vi "Focus Grid Chooser.vi"(10 "SEM Scan Parameters":T2={"X size (um)"=80.0, "Y size (um)"=80.0, "X center (um)"=0.0, "Y center (um)"=0.0, "X size (V)"=3.7333333333333334, "X size auto"=TRUE, "X stig"=[[0.0]], "Y stig"=[[0.0]], "X aln"=[[0.0]], "Y aln"=[[0.0]], "Scan rate (Hz)"=10000000, "Oversampling"=5, "Oversampling auto"=TRUE, "Frame line rampdown ratio"=0.1, "Pixel size (nm)"=8.0, "WD (mm)"=[[3.0]], "X tiles"=1, "Y tiles"=1, "Overlap (um)"=2.0, "Interlaced"=TRUE, "dX (um)"=[0.0], "dY (um)"=[0.0], "Frames"=1} {"dY (um)" format="%.1f"; "dX (um)" format="%.1f"; "Frames" min=1 step=1; "WD (mm)" step=0.001 format="%.4f"; "Y aln" format="%.1f"; "X aln" format="%.1f"; "Y stig" format="%.1f"; "X stig" format="%.1f"; "Overlap (um)" min=0; "Y tiles" min=1; "X tiles" min=1; "X size (um)" format="%.2f"; "Y size (um)" format="%.2f"; "Frame line rampdown ratio" min=0 max=1 step=0.05 format="%.2g"; "X center (um)" step=1 format="%.3f"; "Y center (um)" step=1 format="%.3f"; "X size (V)" format="%_4g"; "Scan rate (Hz)" max=4000000 step=100000 format="%.2e"}, 11 "Focus Index Options":T1={"Keep aspect ratio"=FALSE, "Show Focus Index"=TRUE, "Focus Index primary grid center"=TRUE, "X Grids"=[[1]], "Y Grids"=[[1]], "Primary X index"=[[1]], "Primary Y index"=[[1]]} {"Y Grids" step=2; "X Grids" step=2}) -> (3 "Focus Index Options Out":T1={"Keep aspect ratio"=FALSE, "Show Focus Index"=TRUE, "Focus Index primary grid center"=TRUE, "X Grids"=[[1]], "Y Grids"=[[1]], "Primary X index"=[[1]], "Primary Y index"=[[1]]} {"Y Grids" step=2; "X Grids" step=2})   [LabVIEW 2018]
panel:
  in  "Centered":bool
  out "X Prmry out":u8[][](array[numeric])
  out "Y Prmry out":u8[][](array[numeric])
  out "Tile Y":i32
  out "Tile X":i32
  in  "Tile Grid":bool[][](array[boolean])=[[TRUE, FALSE, FALSE, FALSE, FALSE], [FALSE, FALSE, FALSE, FALSE, FALSE]] caption="Block Face Tile Grid"
  in  "Finished":bool
  out "Y Prmry":u8
  out "X Prmry":u8
  in  "Nx Grids":u8=1 min=1 step=1
  in  "Ny Grids":u8=1 min=1 step=1
  in  "PF Grid":bool[][](array[boolean]) caption="Tile's Primary-Focus Grid"
  # "Grids"
  # "Primary"
  # "Grids"
  # "Primary"
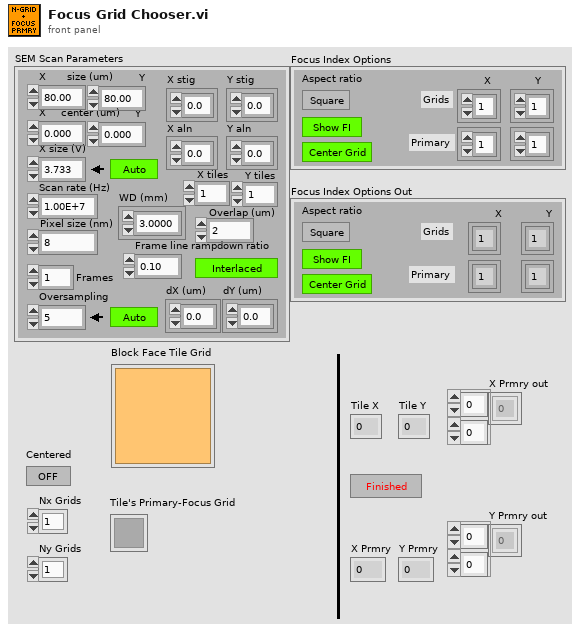
[diagram p1: front panel]
types:
  T1 = cluster{"Keep aspect ratio":bool, "Show Focus Index":bool, "Focus Index primary grid center":bool, "X Grids":u8[][], "Y Grids":u8[][], "Primary X index":u8[][], "Primary Y index":u8[][]}
  T2 = cluster{"X size (um)":sgl, "Y size (um)":sgl, "X center (um)":sgl, "Y center (um)":sgl, "X size (V)":dbl, "X size auto":bool, "X stig":sgl[][], "Y stig":sgl[][], "X aln":sgl[][], "Y aln":sgl[][], "Scan rate (Hz)":u32, "Oversampling":u32, "Oversampling auto":bool, "Frame line rampdown ratio":sgl, "Pixel size (nm)":sgl, "WD (mm)":sgl[][], "X tiles":u8, "Y tiles":u8, "Overlap (um)":sgl, "Interlaced":bool, "dX (um)":sgl[], "dY (um)":sgl[], "Frames":u8}
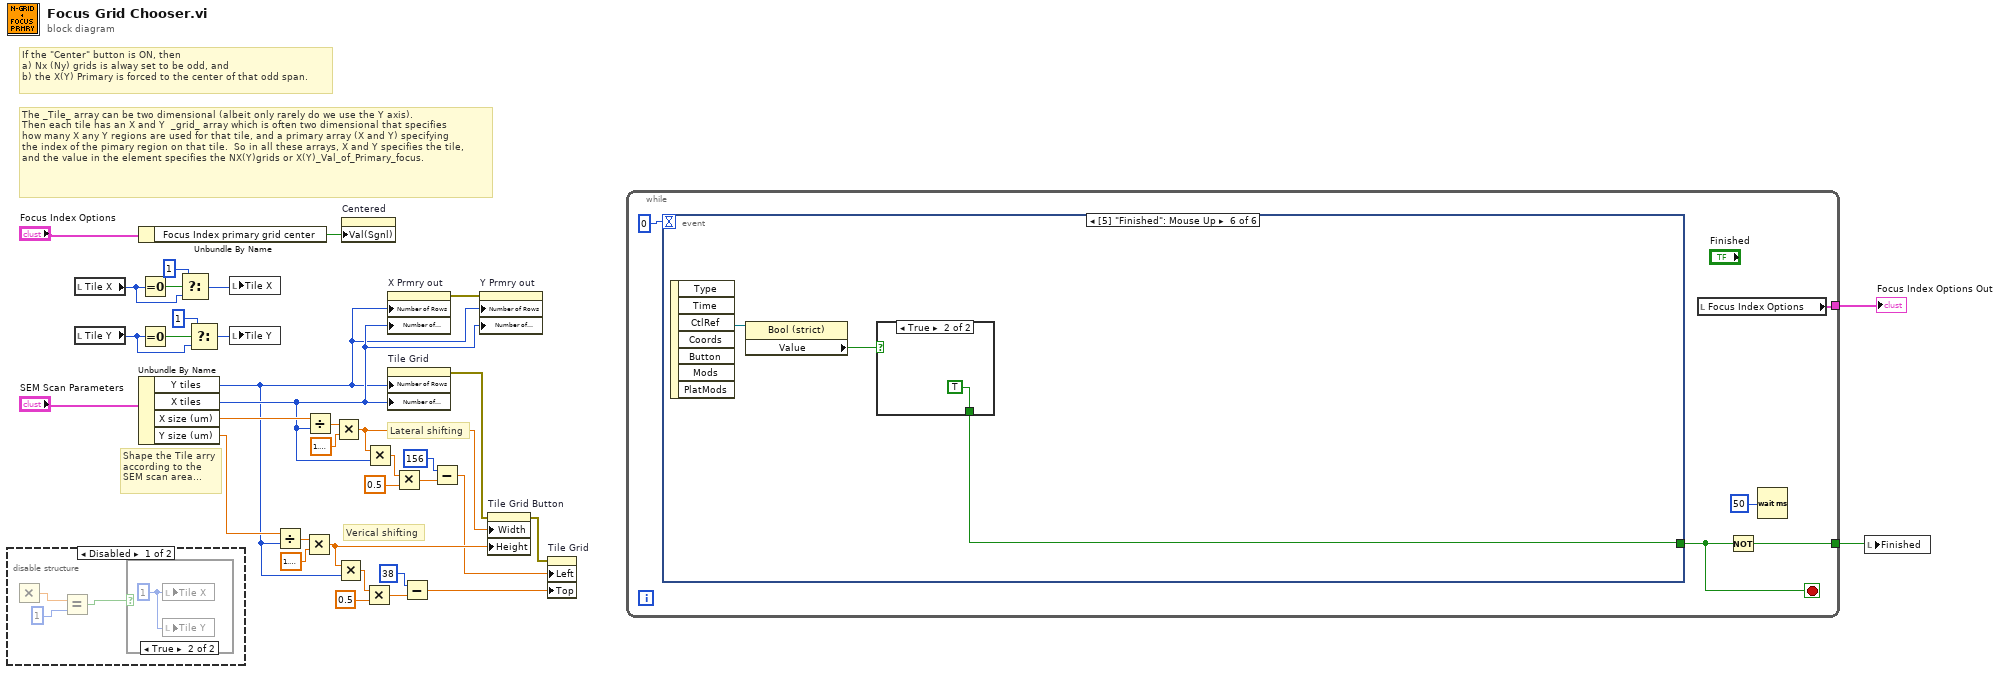
[diagram p0: block diagram]
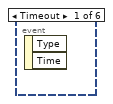
[diagram p4: hidden frame]
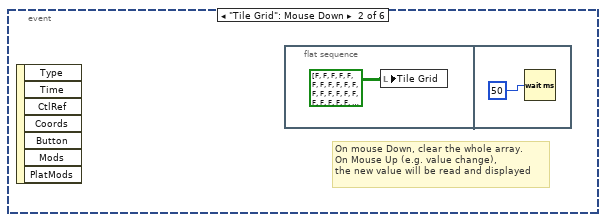
[diagram p5: hidden frame]
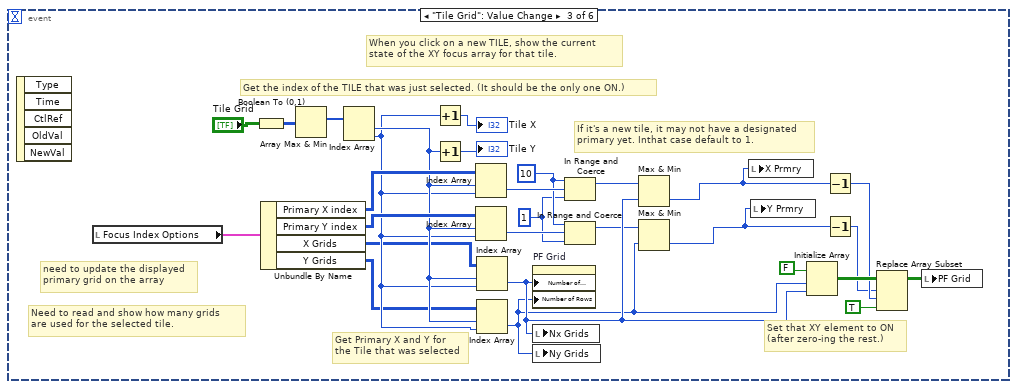
[diagram p6: hidden frame]
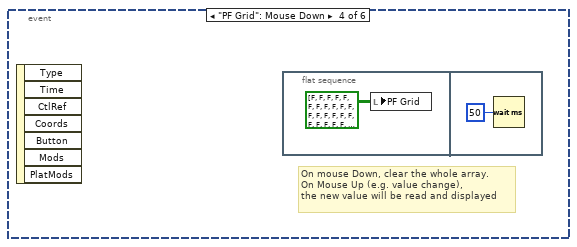
[diagram p7: hidden frame]
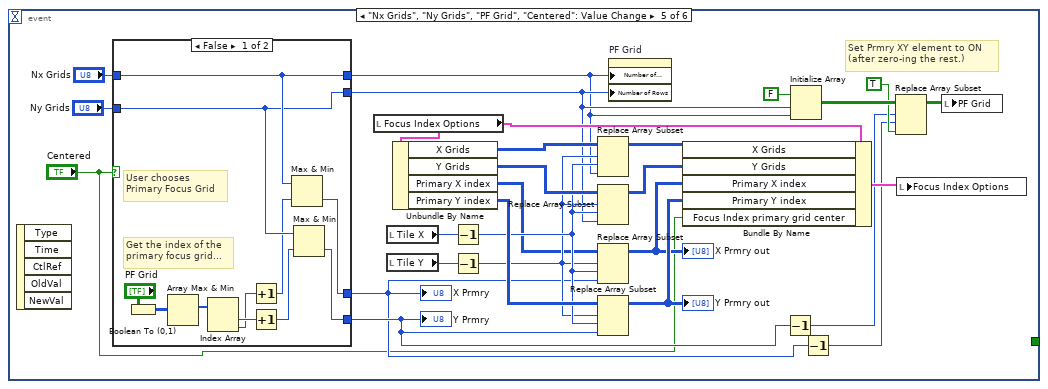
[diagram p8: hidden frame]
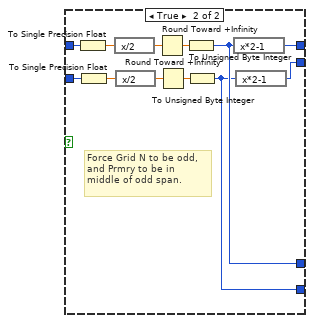
[diagram p9: hidden frame]
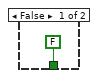
[diagram p10: hidden frame]
diagram:
  # "Shape the Tile arry\naccording to the\nSEM scan area..."
  # "Verical shifting"
  # "Lateral shifting"
  # "If the \"Center\" button is ON, then \na) Nx (Ny) grids is alway set to be odd, and \nb) the X(Y) Primary is forced to the center of that odd span."
  # "The _Tile_ array can be two dimensional (albeit only rarely do we use the Y axis).  \nThen each tile has an X and Y  _grid_ array which is often two dimensional that specifies\nhow many X any Y regions are used for that tile, and a primary array (X and Y) specifying\nthe index of the pimary region on that tile.  So in all these arrays, X and Y specifies the tile, \nand the value in the element specifies the NX(Y)grids or X(Y)_Val_of_Primary_focus."
  n1 = disable-structure shown="Disabled" {
    frame Disabled {
      n2 = Multiply() -> (x*y=w39:dbl)  [unwired: 2 in]
      n3 = Equal?(x=w39, y=u8 1) -> (x = y?=w37:bool)
      n4 = case shown="True" w37 {
        frame False {
        }
        frame True {
          w40 = 1 ("Tile X")
          n5 = local write "Tile X"(w40) -> ()
          n6 = local write "Tile Y"(w40) -> ()
        }
      }
    }
    frame Enabled {
    }
  }
  n7 = local read "Tile X"() -> (w7:i32)
  n8 = local read "Tile Y"() -> (w1:i32)
  n9 = Unbundle By Name("Focus Index Options") -> ("Focus Index primary grid center"=w16:bool)
  n10 = Unbundle By Name("SEM Scan Parameters") -> ("Y tiles"=w10:u8, "X tiles"=w11:u8, "X size (um)"=w34:sgl, "Y size (um)"=w17:sgl)
  n11 = Equal To 0?(x=w7) -> (x = 0?=w8:bool)
  n12 = Equal To 0?(x=w1) -> (x = 0?=w2:bool)
  n13 = Select(t=1, s=w8, f=w7) -> (s? t:f=w5:i32)
  n14 = Select(t=1, s=w2, f=w1) -> (s? t:f=w3:i32)
  n15 = local write "Tile X"(w5) -> ()
  n16 = local write "Tile Y"(w3) -> ()
  n17 = Divide(x=w17, y=w10) -> (x/y=w24:sgl)
  n18 = Multiply(x=w24, y=sgl 1.2) -> (x*y=w21:sgl)
  n19 = Divide(x=w34, y=w11) -> (x/y=w33:sgl)
  n20 = Multiply(x=w33, y=sgl 1.2) -> (x*y=w31:sgl)
  n21 = Multiply(x=w21, y=w10) -> (x*y=w27:sgl)
  n22 = property on="Centered" class="Bool (strict)"("Val(Sgnl)"=w16) -> ()  [unwired: 2 in, 2 out]
  n23 = Multiply(x=w27, y=sgl 0.5 ("x")) -> (x*y=w23:sgl)
  n24 = Multiply(x=w31, y=w11) -> (x*y=w29:sgl)
  n25 = property on="X Prmry out" class="Arr (strict)"("Number of Rows"=w10, "Number of Columns"=w11) -> (error out=w15:errorcluster)  [unwired: 2 in, 1 out]
  n26 = property on="Tile Grid" class="Arr"("Number of Rows"=w10, "Number of Columns"=w11) -> (error out=w28:errorcluster)  [unwired: 2 in, 1 out]
  n27 = Multiply(x=w29, y=sgl 0.5 ("x")) -> (x*y=w35:sgl)
  n28 = Subtract(x=u32 38 ("Button Size:Height"), y=w23) -> (x-y=w18:sgl)
  n29 = Subtract(x=u32 156 ("Button Size:Height"), y=w35) -> (x-y=w19:sgl)
  n30 = property on="Y Prmry out" class="Arr (strict)"(error in=w15, "Number of Rows"=w10, "Number of Columns"=w11) -> ()  [unwired: 1 in, 2 out]
  n31 = property on="Tile Grid Button" class="Bool"(error in=w28, "Width"=w31, "Height"=w21) -> (error out=w20:errorcluster)  [unwired: 1 in, 1 out]
  n32 = property on="Tile Grid" class="Arr"(error in=w20, "Left"=w19, "Top"=w18) -> ()  [unwired: 1 in, 2 out]
  n33 = while {
    tunnel: [w43] -> w12
    tunnel: [w41] -> w9
    stop <- w42 stop-if-true
    n34 = event shown="[5] \"Finished\": Mouse Up" {
      selector: _ -> [_ _ _ _ _ _]
      dyn-events: _ -> [_ _ _ _ _ _]
      timeout: 0 -> [_ _ _ _ _ _]
      tunnel: [_ _ _ _ _ w128] -> w42
      event Timeout {
        n35 = event-data() -> ()  [unwired: 1 in, 2 out]
      }
      event "Tile Grid": Mouse Down {
        # "On mouse Down, clear the whole array.  \nOn Mouse Up (e.g. value change),\nthe new value will be read and displayed"
        n36 = event-data() -> ()  [unwired: 1 in, 7 out]
        n37 = flat-sequence {
          frame #0 {
            n38 = local write "Tile Grid"(bool[][] [[FALSE, FALSE, FALSE, FALSE, FALSE, FALSE, FALSE, FALSE, FALSE, FALSE, FALSE], [FALSE, FALSE, FALSE, FALSE, FALSE, FALSE, FALSE, FALSE, FALSE, FALSE, FALSE], [FALSE, FALSE, FALSE, FALSE, FALSE, FALSE, FALSE, FALSE, FALSE, FALSE, FALSE], [FALSE, FALSE, FALSE, FALSE, FALSE, FALSE, FALSE, FALSE, FALSE, FALSE, FALSE], [FALSE, FALSE, FALSE, FALSE, FALSE, FALSE, FALSE, FALSE, FALSE, FALSE, FALSE], [FALSE, FALSE, FALSE, FALSE, FALSE, FALSE, FALSE, FALSE, FALSE, FALSE, FALSE], [FALSE, FALSE, FALSE, FALSE, FALSE, FALSE, FALSE, FALSE, FALSE, FALSE, FALSE], [FALSE, FALSE, FALSE, FALSE, FALSE, FALSE, FALSE, FALSE, FALSE, FALSE, FALSE], [FALSE, FALSE, FALSE, FALSE, FALSE, FALSE, FALSE, FALSE, FALSE, FALSE, FALSE], [FALSE, FALSE, FALSE, FALSE, FALSE, FALSE, FALSE, FALSE, FALSE, FALSE, FALSE], [FALSE, FALSE, FALSE, FALSE, FALSE, FALSE, FALSE, FALSE, FALSE, FALSE, FALSE]] ("Tile Primary-Focus Grid")) -> ()
          }
          frame #1 {
            n39 = Wait (ms)(milliseconds to wait=u32 50) -> ()  [unwired: 1 out]
          }
        }
      }
      event "Tile Grid": Value Change {
        w54 = u8 1 ("lower limit")
        w55 = u8 10 ("upper limit")
        # "If it's a new tile, it may not have a designated\nprimary yet. Inthat case default to 1."
        # "Need to read and show how many grids \nare used for the selected tile."
        # "When you click on a new TILE, show the current\nstate of the XY focus array for that tile."
        # "Set that XY element to ON\n(after zero-ing the rest.)"
        # "Get Primary X and Y for\nthe Tile that was selected"
        # "need to update the displayed\nprimary grid on the array"
        # "Get the index of the TILE that was just selected. (It should be the only one ON.)"
        n40 = event-data() -> ()  [unwired: 1 in, 5 out]
        n41 = local read "Focus Index Options"() -> (w70:T1)
        n42 = Boolean To (0,1)(Boolean="Tile Grid") -> (0, 1=w74:i16[][])
        n43 = Unbundle By Name(w70) -> ("Primary X index"=w69:u8[][], "Primary Y index"=w68:u8[][], "X Grids"=w59:u8[][], "Y Grids"=w58:u8[][])
        n44 = Array Max & Min(array=w74) -> (max index (indices)=w73:i32[])  [unwired: 3 out]
        n45 = Index Array(array=w73) -> (element #1=w61:i32, element #2=w60:i32)  [unwired: 2 in]
        n46 = Increment(x=w60) -> (x+1=→"Tile X":i32)
        n47 = Increment(x=w61) -> (x+1=→"Tile Y":i32)
        n48 = Index Array(array=w69, index (row)=w61, index (col)=w60) -> (element=w57:u8)
        n49 = Index Array(array=w68, index (row)=w61, index (col)=w60) -> (element=w56:u8)
        n50 = Index Array(array=w59, index (row)=w61, index (col)=w60) -> (element=w53:u8)
        n51 = Index Array(array=w58, index (row)=w61, index (col)=w60) -> (element=w48:u8)
        n52 = property on="PF Grid" class="Arr"("Number of Columns"=w53, "Number of Rows"=w48) -> ()  [unwired: 2 in, 2 out]
        n53 = local write "Nx Grids"(w53) -> ()
        n54 = local write "Ny Grids"(w48) -> ()
        n55 = In Range and Coerce(upper limit=w55, x=w57, lower limit=w54) -> (coerced(x)=w52:u8)  [unwired: 1 out]
        n56 = In Range and Coerce(upper limit=w55, x=w56, lower limit=w54) -> (coerced(x)=w50:u8)  [unwired: 1 out]
        n57 = Max & Min(x=w52, y=w53) -> (min(x,y)=w51:u8)  [unwired: 1 out]
        n58 = Max & Min(x=w50, y=w48) -> (min(x,y)=w49:u8)  [unwired: 1 out]
        n59 = local write "X Prmry"(w51) -> ()
        n60 = local write "Y Prmry"(w49) -> ()
        n61 = Initialize Array(FALSE, w48, w53) -> (w71:bool[][])
        n62 = Decrement(x=w51) -> (x-1=w63:u8)
        n63 = Decrement(x=w49) -> (x-1=w62:u8)
        n64 = Replace Array Subset(array=w71, new element=TRUE, index (row)=w62, index (col)=w63) -> (w64:bool[][])
        n65 = local write "PF Grid"(w64) -> ()
      }
      event "PF Grid": Mouse Down {
        # "On mouse Down, clear the whole array.  \nOn Mouse Up (e.g. value change),\nthe new value will be read and displayed"
        n66 = event-data() -> ()  [unwired: 1 in, 7 out]
        n67 = flat-sequence {
          frame #0 {
            n68 = local write "PF Grid"(bool[][] [[FALSE, FALSE, FALSE, FALSE, FALSE, FALSE, FALSE, FALSE, FALSE, FALSE, FALSE], [FALSE, FALSE, FALSE, FALSE, FALSE, FALSE, FALSE, FALSE, FALSE, FALSE, FALSE], [FALSE, FALSE, FALSE, FALSE, FALSE, FALSE, FALSE, FALSE, FALSE, FALSE, FALSE], [FALSE, FALSE, FALSE, FALSE, FALSE, FALSE, FALSE, FALSE, FALSE, FALSE, FALSE], [FALSE, FALSE, FALSE, FALSE, FALSE, FALSE, FALSE, FALSE, FALSE, FALSE, FALSE], [FALSE, FALSE, FALSE, FALSE, FALSE, FALSE, FALSE, FALSE, FALSE, FALSE, FALSE], [FALSE, FALSE, FALSE, FALSE, FALSE, FALSE, FALSE, FALSE, FALSE, FALSE, FALSE], [FALSE, FALSE, FALSE, FALSE, FALSE, FALSE, FALSE, FALSE, FALSE, FALSE, FALSE], [FALSE, FALSE, FALSE, FALSE, FALSE, FALSE, FALSE, FALSE, FALSE, FALSE, FALSE], [FALSE, FALSE, FALSE, FALSE, FALSE, FALSE, FALSE, FALSE, FALSE, FALSE, FALSE], [FALSE, FALSE, FALSE, FALSE, FALSE, FALSE, FALSE, FALSE, FALSE, FALSE, FALSE]] ("Tile Primary-Focus Grid")) -> ()
          }
          frame #1 {
            n69 = Wait (ms)(milliseconds to wait=u32 50) -> ()  [unwired: 1 out]
          }
        }
      }
      event "Nx Grids", "Ny Grids", "PF Grid", "Centered": Value Change {
        # "Set Prmry XY element to ON\n(after zero-ing the rest.)"
        n70 = event-data() -> ()  [unwired: 1 in, 5 out]
        n71 = case shown="False" "Centered" {
          tunnel: [w109 w118] -> w86
          tunnel: [w110 w126] -> w85
          tunnel: [w105 w117] -> w80
          tunnel: [w106 w116] -> w82
          tunnel: "Nx Grids" -> [w110 w123]
          tunnel: "Ny Grids" -> [w109 w119]
          frame False {
            # "User chooses \nPrimary Focus Grid"
            # "Get the index of the\nprimary focus grid..."
            n72 = Boolean To (0,1)(Boolean="PF Grid") -> (0, 1=w115:i16[][])
            n73 = Array Max & Min(array=w115) -> (max index (indices)=w114:i32[])  [unwired: 3 out]
            n74 = Index Array(array=w114) -> (element #1=w112:i32, element #2=w111:i32)  [unwired: 2 in]
            n75 = Increment(x=w111) -> (x+1=w108:i32)
            n76 = Increment(x=w112) -> (x+1=w107:i32)
            n77 = Max & Min(x=w110, y=w108) -> (min(x,y)=w105:i32)  [unwired: 1 out]
            n78 = Max & Min(x=w109, y=w107) -> (min(x,y)=w106:i32)  [unwired: 1 out]
          }
          frame True {
            # "Force Grid N to be odd,\nand Prmry to be in\nmiddle of odd span."
            n79 = To Single Precision Float(number=w123) -> (single precision float=w125:sgl)
            n80 = To Single Precision Float(number=w119) -> (single precision float=w121:sgl)
            n81 = expression code="x/2"(w125) -> (w127:sgl)
            n82 = expression code="x/2"(w121) -> (w120:sgl)
            n83 = Round Toward +Infinity(x=w127) -> (ceil(x): smallest int >= x=w124:sgl)
            n84 = Round Toward +Infinity(x=w120) -> (ceil(x): smallest int >= x=w122:sgl)
            n85 = To Unsigned Byte Integer(number=w124) -> (unsigned 8bit integer=w117:u8)
            n86 = To Unsigned Byte Integer(number=w122) -> (unsigned 8bit integer=w116:u8)
            n87 = expression code="x*2-1"(w117) -> (w126:u8)
            n88 = expression code="x*2-1"(w116) -> (w118:u8)
          }
        }
        "X Prmry" <- w80
        "Y Prmry" <- w82
        n89 = local read "Focus Index Options"() -> (w98:T1)
        n90 = local read "Tile X"() -> (w99:i32)
        n91 = local read "Tile Y"() -> (w100:i32)
        n92 = Unbundle By Name(w98) -> ("X Grids"=w103:u8[][], "Y Grids"=w101:u8[][], "Primary X index"=w93:u8[][], "Primary Y index"=w96:u8[][])
        n93 = Decrement(x=w99) -> (x-1=w95:i32)
        n94 = Decrement(x=w100) -> (x-1=w94:i32)
        n95 = Replace Array Subset(array=w103, new element=w85, index (row)=w94, index (col)=w95) -> (w102:u8[][])
        n96 = Replace Array Subset(array=w101, new element=w86, index (row)=w94, index (col)=w95) -> (w97:u8[][])
        n97 = Replace Array Subset(array=w93, new element=w80, index (row)=w94, index (col)=w95) -> (w91:u8[][])
        "X Prmry out" <- w91
        n98 = Replace Array Subset(array=w96, new element=w82, index (row)=w94, index (col)=w95) -> (w92:u8[][])
        "Y Prmry out" <- w92
        n99 = property on="PF Grid" class="Arr"("Number of Columns"=w85, "Number of Rows"=w86) -> ()  [unwired: 2 in, 2 out]
        n100 = Bundle By Name(cluster=w98, "X Grids"=w102, "Y Grids"=w97, "Primary X index"=w91, "Primary Y index"=w92, "Focus Index primary grid center"="Centered") -> (w104:T1)
        n101 = Decrement(x=w82) -> (x-1=w81:i32)
        n102 = Initialize Array(FALSE, w86, w85) -> (w88:bool[][])
        n103 = Decrement(x=w80) -> (x-1=w79:i32)
        n104 = Replace Array Subset(array=w88, new element=TRUE, index (row)=w81, index (col)=w79) -> (w83:bool[][])
        n105 = local write "Focus Index Options"(w104) -> ()
        n106 = local write "PF Grid"(w83) -> ()
      }
      event "Finished": Mouse Up {
        n107 = event-data() -> ("CtlRef"=w130:refnum<vi>)  [unwired: 1 in, 6 out]
        n108 = property class="Bool (strict)"(reference=w130) -> ("Value"=w129:bool)  [unwired: 1 in, 2 out]
        n109 = case shown="True" w129 {
          tunnel: [FALSE ("Finished") TRUE ("Finished")] -> w128
          frame False {
          }
          frame True {
          }
        }
      }
    }
    n110 = local read "Focus Index Options"() -> (w43:T1)
    n111 = Not(x=w42) -> (.not. x?=w41:bool)
    n112 = Wait (ms)(milliseconds to wait=u32 50) -> ()  [unwired: 1 out]
  }
  "Focus Index Options Out" <- w12
  n113 = local write "Finished"(w9) -> ()
